vi "Acoustic Frequency Response Stepped Sine.vi"(0 "TSM context":T2, 5 "Sweep Configuration":T1[](array[typedef]), 7 "Duration in Cycles? (F)":bool, 11 "error in (no error)":errorcluster) -> (4 "DUT Measurements":dbl[][](array[numeric]), 6 "RefMic Measurements":dbl[][](array[numeric]), 15 "error out":errorcluster)   [LabVIEW 2020]
uses:
  <vilib>/NI_TestStand_SemiconductorModule/NI_TestStand_Semiconductor_Module.lvlibp/PinMap/General/SemiconductorModuleContext.ctl
  Typedefs/Acoustic Sweep Config Cluster.ctl
  8f7c203c-f693-4b0c-9260-738b7318b847.vi
  2f406ff7-c9b3-4e57-b80f-89e5fed583d8.vi
  e2d7146d-6857-41e7-9267-930fdada05f6.vi
  8d1380fc-7ee0-47bb-9c65-33dd6d969f66.vi
  8492cc62-2198-43ea-8a81-0fb3a5915e80.vi
  8f7c203c-f693-4b0c-9260-738b7318b847.vi/8b04a85c-40a8-485d-9537-76eecc64180b.vi
  <vilib>/NI_TestStand_SemiconductorModule/NI_TestStand_Semiconductor_Module.lvlibp
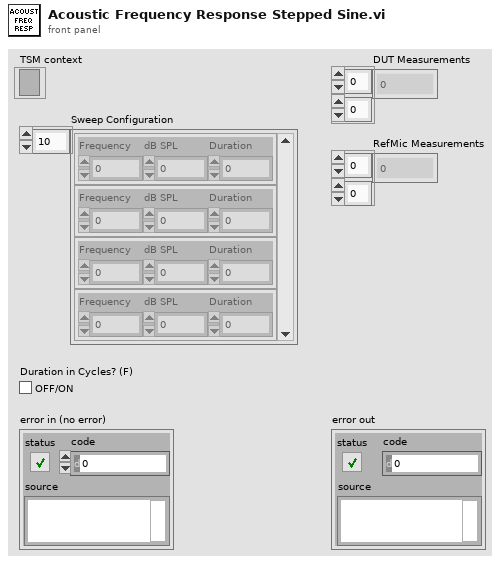
[diagram p1: front panel]
types:
  T1 = typedef "Acoustic Sweep Config Cluster.ctl" = cluster{"Frequency":dbl, "dB SPL":dbl, "Duration":dbl}
  T2 = typedef "NI_TestStand_Semiconductor_Module.lvlibp/SemiconductorModuleContext.ctl" = refnum<k7>
  T3 = typedef "TSM DAQmx Multi-Task.ctl" = cluster{"Pin Query Context":refnum<class "MultiplePinMultipleSessionQueryContext.lvclass">, "SSC":T4[], "Site Numbers":i32[], "Pins":tag[]}
  T4 = typedef "SSC DAQmx.ctl" = cluster{"DAQmx Task ":refnum<k21>, "Channels":string, "Channel Lists":string}
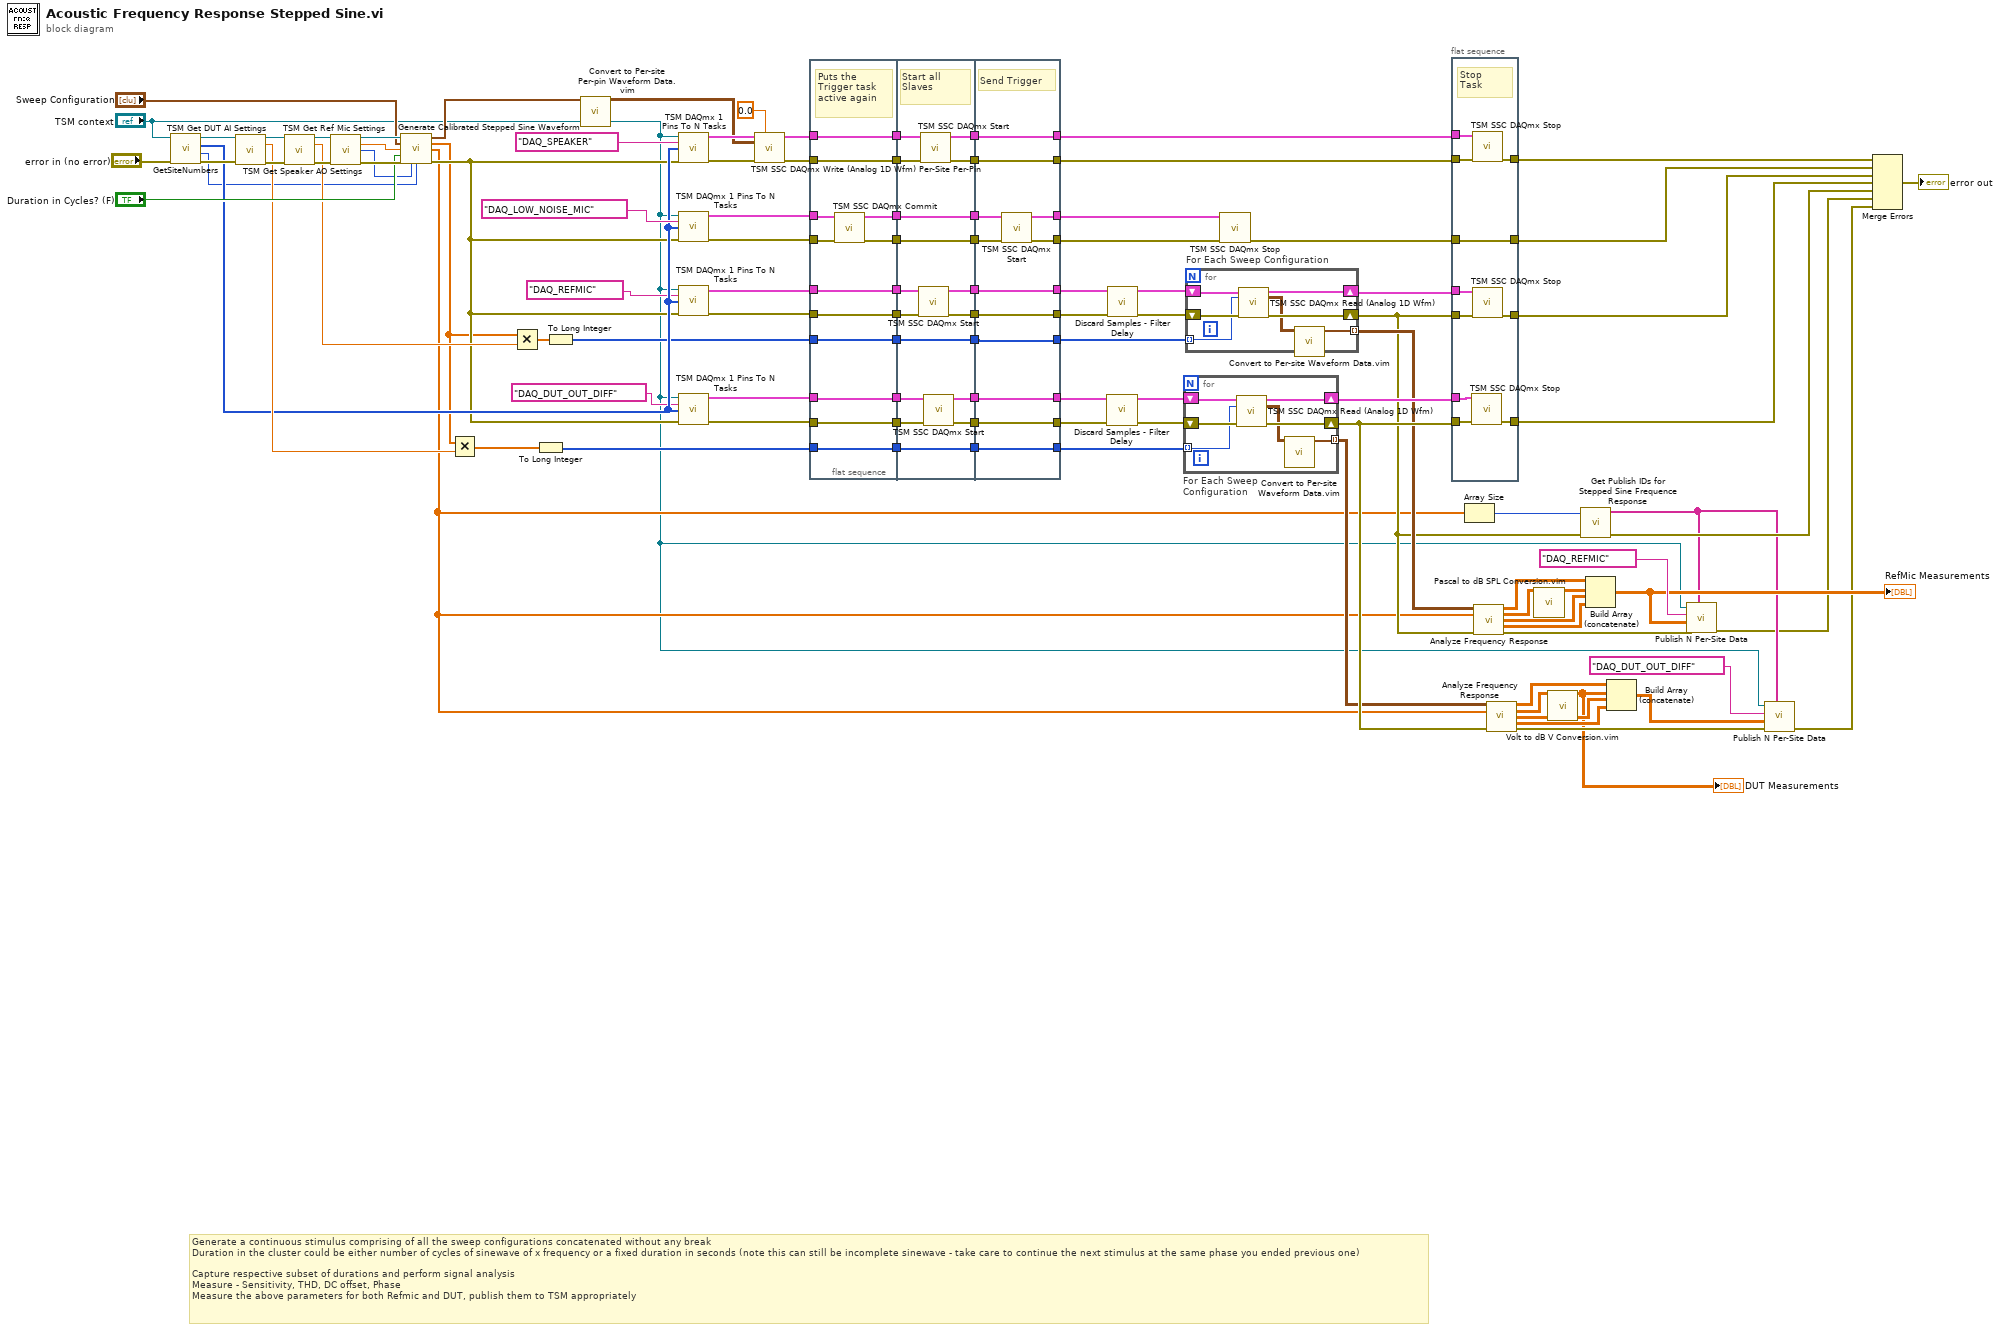
[diagram p0: block diagram]
diagram:
  # "Generate a continuous stimulus comprising of all the sweep configurations concatenated without any break\nDuration in the cluster could be either number of cycles of sinewave of x frequency or a fixed duration in seconds (note this can still be incomplete sinewave - take care to continue the next stimulus at the same phase you ended previous one)\n\nCapture respective subset of durations and perform signal analysis\nMeasure - Sensitivity, THD, DC offset, Phase\nMeasure the above parameters for both Refmic and DUT, publish them to TSM appropriately"
  n1 = call <vilib>:"GetSiteNumbers.vi"("error in (no error)"="error in (no error)", "Semiconductor Module Context"="TSM context") -> ("error out"=w109:errorcluster, "Number Of Sites"=w33:i32, "Site Numbers"=w80:i32[], "Semiconductor Module Context Out"=w108:T2)  [unwired: 6 in]
  n2 = call "TSM Get DUT AI Settings.vi"("TSM context"=w108, "error in (no error)"=w109) -> ("TSM context Out"=w105:T2, "Sampling Rate (Hz)"=w85:dbl, "error out"=w107:errorcluster)  [unwired: 9 in, 2 out]
  n3 = call "TSM Get Ref Mic Settings.vi"("TSM context"=w105, "error in (no error)"=w107) -> ("TSM context Out"=w104:T2, "Sampling Rate (Hz)"=w86:dbl, "error out"=w106:errorcluster)  [unwired: 8 in, 3 out]
  n4 = call "TSM Get Speaker AO Settings.vi"("TSM context"=w104, "error in (no error)"=w106) -> ("TSM context Out"=w90:T2, "Sampling Rate (Hz)"=w88:dbl, "Samples per channel"=w32:i32, "error out"=w91:errorcluster)  [unwired: 9 in, 1 out]
  n5 = call "Generate Calibrated Stepped Sine Waveform.vi"("TSM context"=w90, "Sweep Configuration"="Sweep Configuration", "Sample rate"=w88, "Duration in Cycles? (F)"="Duration in Cycles? (F)", "error in (no error)"=w91, "Total Expected Samples"=w32, "Number Of Sites"=w33) -> ("PerSite Waveform"=w42:waveform(dbl)[], "Capture Duration"=w78:dbl[], "Frequency"=w22:dbl[], "error out"=w79:errorcluster)  [unwired: 5 in]
  n6 = Multiply(x=w78, y=w85) -> (x*y=w83:dbl[])
  n7 = Multiply(x=w78, y=w86) -> (x*y=w84:dbl[])
  n8 = To Long Integer(number=w83) -> (32bit integer=w47:i32[])
  n9 = To Long Integer(number=w84) -> (32bit integer=w53:i32[])
  n10 = call "Convert to Per-site Per-pin Waveform Data.vim"("Waveform In"=w42) -> ("Per Site Per Pin Waveform Out"=w41:waveform(dbl)[][])  [unwired: 14 in]
  n11 = call "TSM DAQmx 1 Pins To N Tasks.vi"("TSM context"="TSM context", "Pins"=tag "DAQ_SPEAKER", "Site Numbers"=w80, "error in"=w79) -> ("DAQ TSM Out"=w73:T3, "error out"=w75:errorcluster)  [unwired: 10 in]
  n12 = call "TSM DAQmx 1 Pins To N Tasks.vi"("TSM context"="TSM context", "Pins"=tag "DAQ_LOW_NOISE_MIC", "Site Numbers"=w80, "error in"=w79) -> ("DAQ TSM Out"=w69:T3, "error out"=w70:errorcluster)  [unwired: 10 in]
  n13 = call "TSM DAQmx 1 Pins To N Tasks.vi"("TSM context"="TSM context", "Pins"=tag "DAQ_REFMIC", "Site Numbers"=w80, "error in"=w79) -> ("DAQ TSM Out"=w61:T3, "error out"=w62:errorcluster)  [unwired: 10 in]
  n14 = call "TSM DAQmx 1 Pins To N Tasks.vi"("TSM context"="TSM context", "Pins"=tag "DAQ_DUT_OUT_DIFF", "Site Numbers"=w80, "error in"=w79) -> ("DAQ TSM Out"=w63:T3, "error out"=w64:errorcluster)  [unwired: 10 in]
  n15 = call "TSM SSC DAQmx Write (Analog 1D Wfm) Per-Site Per-Pin.vi"("DAQ TSM in"=w73, "Idle Channel Value (0)"=0.0, "Per-Site Per-Pin Waveforms in"=w41, "error in"=w75) -> ("DAQ TSM Out"=w71:T3, "error out"=w72:errorcluster)  [unwired: 10 in]
  n16 = flat-sequence {
    tunnel: w71 -> [w118]
    tunnel: w72 -> [w119]
    tunnel: w61 -> [w120]
    tunnel: w62 -> [w121]
    tunnel: [w121] -> w103
    tunnel: [w120] -> w102
    tunnel: [w119] -> w101
    tunnel: [w118] -> w100
    tunnel: w70 -> [w117]
    tunnel: w69 -> [w116]
    tunnel: [w115] -> w99
    tunnel: [w114] -> w98
    tunnel: [w112] -> w66
    tunnel: [w113] -> w65
    tunnel: w63 -> [w113]
    tunnel: w64 -> [w112]
    tunnel: w53 -> [w111]
    tunnel: [w111] -> w52
    tunnel: w47 -> [w110]
    tunnel: [w110] -> w46
    tunnel: w103 -> [w133]
    tunnel: w102 -> [w132]
    tunnel: w101 -> [w137]
    tunnel: w100 -> [w135]
    tunnel: w99 -> [w129]
    tunnel: w98 -> [w128]
    tunnel: [w136] -> w97
    tunnel: [w134] -> w96
    tunnel: [w130] -> w95
    tunnel: [w131] -> w94
    tunnel: [w129] -> w93
    tunnel: [w128] -> w92
    tunnel: [w127] -> w68
    tunnel: [w126] -> w67
    tunnel: w66 -> [w124]
    tunnel: w65 -> [w125]
    tunnel: w52 -> [w123]
    tunnel: [w123] -> w51
    tunnel: w46 -> [w122]
    tunnel: [w122] -> w44
    tunnel: [w146] -> w6
    tunnel: [w147] -> w56
    tunnel: [w148] -> w58
    tunnel: [w149] -> w59
    tunnel: w97 -> [w149]
    tunnel: w96 -> [w148]
    tunnel: w95 -> [w147]
    tunnel: w94 -> [w146]
    tunnel: w93 -> [w145]
    tunnel: w92 -> [w144]
    tunnel: [w143] -> w54
    tunnel: [w142] -> w60
    tunnel: [w141] -> w3
    tunnel: [w140] -> w49
    tunnel: w68 -> [w140]
    tunnel: w67 -> [w141]
    tunnel: [w139] -> w50
    tunnel: w51 -> [w139]
    tunnel: [w138] -> w45
    tunnel: w44 -> [w138]
    frame #0 {
      # "Puts the Trigger task active again"
      n17 = call "TSM SSC DAQmx Commit.vi"("TSM DAQmx In"=w116, "error in (no error)"=w117) -> ("TSM DAQmx Out"=w114:T3, "error out"=w115:errorcluster)  [unwired: 12 in]
    }
    frame #1 {
      # "Start all Slaves"
      n18 = call "TSM SSC DAQmx Start.vi"("TSM DAQmx In"=w132, "error in (no error)"=w133) -> ("TSM DAQmx Out"=w131:T3, "error out"=w130:errorcluster)  [unwired: 12 in]
      n19 = call "TSM SSC DAQmx Start.vi"("TSM DAQmx In"=w135, "error in (no error)"=w137) -> ("TSM DAQmx Out"=w134:T3, "error out"=w136:errorcluster)  [unwired: 12 in]
      n20 = call "TSM SSC DAQmx Start.vi"("TSM DAQmx In"=w125, "error in (no error)"=w124) -> ("TSM DAQmx Out"=w126:T3, "error out"=w127:errorcluster)  [unwired: 12 in]
    }
    frame #2 {
      # "Send Trigger"
      n21 = call "TSM SSC DAQmx Start.vi"("TSM DAQmx In"=w144, "error in (no error)"=w145) -> ("TSM DAQmx Out"=w143:T3, "error out"=w142:errorcluster)  [unwired: 12 in]
    }
  }
  n22 = call "Discard Samples - Filter Delay.vi"("DAQ TSM in"=w3, "error in"=w49) -> ("DAQ TSM Out"=w2:T3, "error out"=w4:errorcluster)  [unwired: 12 in]
  n23 = call "Discard Samples - Filter Delay.vi"("DAQ TSM in"=w6, "error in"=w56) -> ("DAQ TSM Out"=w5:T3, "error out"=w7:errorcluster)  [unwired: 12 in]
  n24 = for "For Each Sweep Configuration" {
    shift-right: [w154] -> w43
    shift-left: w4 -> [w156]
    shift-right: [w153] -> w48
    shift-left: w2 -> [w155]
    tunnel: w45 -> [w152] mode=indexing
    tunnel: [w150] -> w39 mode=indexing
    n25 = call "TSM SSC DAQmx Read (Analog 1D Wfm).vi"("DAQ TSM in"=w155, "Samples to read"=w152, "error in"=w156) -> ("DAQ TSM Out"=w153:T3, "Per-Site Per-Pin Waveforms Out"=w151:waveform(dbl)[][], "error out"=w154:errorcluster)  [unwired: 10 in]
    n26 = call "Convert to Per-site Waveform Data.vim"("Per-Site Per-Pin Waveform In"=w151) -> ("Per-Site Waveform Out"=w150:waveform(dbl)[])  [unwired: 14 in]
  }
  n27 = for "For Each Sweep Configuration" {
    shift-right: [w161] -> w24
    shift-left: w7 -> [w163]
    shift-right: [w160] -> w55
    shift-left: w5 -> [w162]
    tunnel: w50 -> [w159] mode=indexing
    tunnel: [w157] -> w40 mode=indexing
    n28 = call "TSM SSC DAQmx Read (Analog 1D Wfm).vi"("DAQ TSM in"=w162, "Samples to read"=w159, "error in"=w163) -> ("DAQ TSM Out"=w160:T3, "Per-Site Per-Pin Waveforms Out"=w158:waveform(dbl)[][], "error out"=w161:errorcluster)  [unwired: 10 in]
    n29 = call "Convert to Per-site Waveform Data.vim"("Per-Site Per-Pin Waveform In"=w158) -> ("Per-Site Waveform Out"=w157:waveform(dbl)[])  [unwired: 14 in]
  }
  n30 = call "TSM SSC DAQmx Stop.vi"("TSM DAQmx In"=w54, "error in (no error)"=w60) -> ("error out"=w57:errorcluster)  [unwired: 12 in, 1 out]
  n31 = flat-sequence {
    tunnel: w58 -> [w173]
    tunnel: w59 -> [w172]
    tunnel: w48 -> [w171]
    tunnel: w43 -> [w170]
    tunnel: [w169] -> w35
    tunnel: [w168] -> w38
    tunnel: w57 -> [w167]
    tunnel: [w167] -> w37
    tunnel: w24 -> [w164]
    tunnel: w55 -> [w165]
    tunnel: [w164] -> _
    tunnel: [w166] -> w36
    frame #0 {
      # "Stop \nTask"
      n32 = call "TSM SSC DAQmx Stop.vi"("TSM DAQmx In"=w171, "error in (no error)"=w170) -> ("error out"=w169:errorcluster)  [unwired: 12 in, 1 out]
      n33 = call "TSM SSC DAQmx Stop.vi"("TSM DAQmx In"=w173, "error in (no error)"=w172) -> ("error out"=w168:errorcluster)  [unwired: 12 in, 1 out]
      n34 = call "TSM SSC DAQmx Stop.vi"("TSM DAQmx In"=w165, "error in (no error)"=w164) -> ("error out"=w166:errorcluster)  [unwired: 12 in, 1 out]
    }
  }
  n35 = Array Size(array=w22) -> (size(s)=w23:i32)
  n36 = call "Analyze Frequency Response.vi"("Per-Frequency Per-Site Waveform In"=w40, "Frequency (Hz)"=w22, "error in (no error)"=w24) -> ("DC values(V)"=w31:dbl[][], "detected amplitudes(Unit Peak)"=w28:dbl[][], "detected phases (deg)"=w29:dbl[][], "THD(%)"=w30:dbl[][], "error out"=w21:errorcluster)  [unwired: 8 in]
  n37 = call "Analyze Frequency Response.vi"("Per-Frequency Per-Site Waveform In"=w39, "Frequency (Hz)"=w22, "error in (no error)"=w43) -> ("DC values(V)"=w16:dbl[][], "detected amplitudes(Unit Peak)"=w17:dbl[][], "detected phases (deg)"=w18:dbl[][], "THD(%)"=w19:dbl[][], "error out"=w20:errorcluster)  [unwired: 8 in]
  n38 = call "Pascal to dB SPL Conversion.vim"("Pascals"=w28) -> ("dbSPL"=w27:dbl[][])  [unwired: 14 in]
  n39 = call "Volt to dB V Conversion.vim"("Voltage"=w17) -> ("dB V"=w1:dbl[][])  [unwired: 14 in]
  "DUT Measurements" <- w1
  n40 = call "Get Publish IDs for Stepped Sine Frequence Response.vi"("Error In"=w24, "No of  Sweep Configurations"=w23) -> ("Error Out"=w12:errorcluster, "Publish IDs"=w11:tag[])  [unwired: 8 in]
  n41 = Build Array (concatenate)(w31, w27, w29, w30) -> (w25:dbl[][])
  "RefMic Measurements" <- w25
  n42 = Build Array (concatenate)(w16, w1, w18, w19) -> (w15:dbl[][])
  n43 = call "Publish N Per-Site Data.vi"("Published Data Id"=w11, "error in (no error)"=w21, "Data In"=w25, "Pin"=tag "DAQ_REFMIC" ("Pins"), "Semiconductor Module Context"="TSM context") -> ("error out"=w10:errorcluster)  [unwired: 5 in, 1 out]
  n44 = call "Publish N Per-Site Data.vi"("Published Data Id"=w11, "error in (no error)"=w20, "Data In"=w15, "Pin"=tag "DAQ_DUT_OUT_DIFF" ("Pins"), "Semiconductor Module Context"="TSM context") -> ("error out"=w9:errorcluster)  [unwired: 5 in, 1 out]
  n45 = Merge Errors(w38, w37, w36, w35, w12, w10, w9) -> (→"error out":errorcluster)
